vi "OmegaOutput.vi"(8 "error in (no error)":errorcluster, 10 "String":string) -> (0 "error out":errorcluster, 2 "Cluster":cluster{"omega":sgl, "current":sgl})   [LabVIEW 2021]
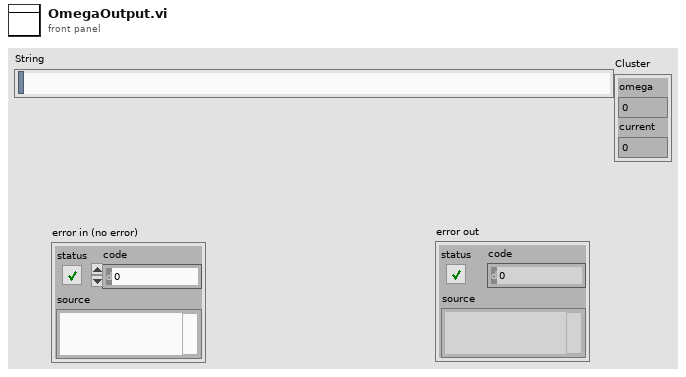
[diagram p1: front panel]
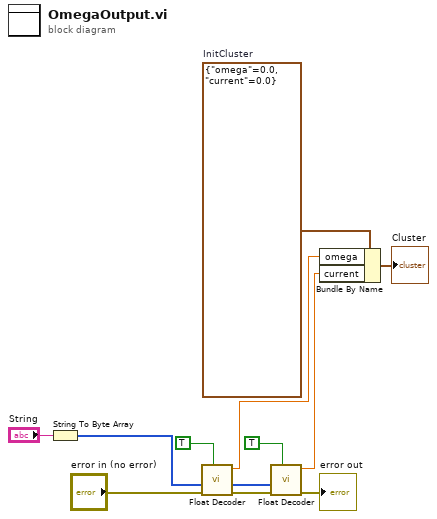
[diagram p0: block diagram]
diagram:
  w11 = cluster{"omega":sgl, "current":sgl} {"omega"=0.0, "current"=0.0}  # InitCluster
  n1 = String To Byte Array(string="String") -> (unsigned byte array=w6:u8[])
  n2 = call "Float Decoder.vi"("Optional"=TRUE, "error in (no error)"="error in (no error)", "Array"=w6) -> ("error out"=w2:errorcluster, "array w/ subset deleted"=w3:u8[], "Float"=w8:sgl)  [unwired: 5 in, 1 out]
  n3 = call "Float Decoder.vi"("Optional"=TRUE, "error in (no error)"=w2, "Array"=w3) -> ("error out"=→"error out":errorcluster, "Float"=w4:sgl)  [unwired: 5 in, 2 out]
  n4 = Bundle By Name(cluster=w11, "omega"=w8, "current"=w4) -> (→"Cluster":cluster{"omega":sgl, "current":sgl})
